vi "tcplink-client -- test.vi"() -> ()   [LabVIEW 2020]
uses:
  publisher action.ctl
  sparkle.ctl
panel:
  in  "millisecond multiple":u32=100
  in  "Stop":bool
  out "Gamma":dbl
  out "frequency":dbl
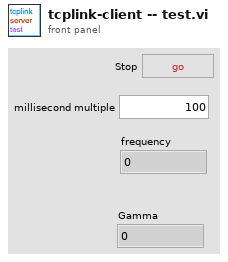
[diagram p1: front panel]
types:
  T1 = typedef "publisher action.ctl" = enum16{"set", "get", "init", "check"}
  T2 = typedef "sparkle.ctl" = cluster{"units":string, "data":dbl}
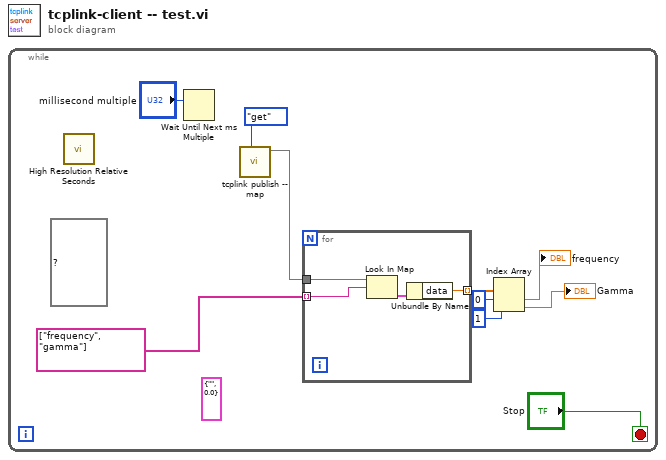
[diagram p0: block diagram]
diagram:
  n1 = while {
    stop <- "Stop" stop-if-true
    (unwired) T2 {"units"="", "data"=0.0} ("sparkle")
    (unwired) map{string, T2} {} ("sparkle map IN")
    n2 = call <vilib>:"High Resolution Relative Seconds.vi"() -> ()  [unwired: 1 out]
    n3 = Wait Until Next ms Multiple(millisecond multiple="millisecond multiple") -> ()  [unwired: 1 out]
    n4 = call "tcplink publish -- map.vi"("publisher action"=publisher_action."get") -> ("sparkle map OUT"=w6:map{string, T2})  [unwired: 10 in]
    n5 = for {
      tunnel: string[] ["frequency", "gamma"] ("string array IN") -> [w13] mode=indexing
      tunnel: w6 -> [w14]
      tunnel: [w11] -> w5 mode=indexing
      n6 = Look In Map(map=w14, key=w13) -> (value=w12:T2)  [unwired: 1 in, 1 out]
      n7 = Unbundle By Name(w12) -> ("data"=w11:dbl)
    }
    n8 = Index Array(array=w5, index #1=0 ("index"), index #2=1 ("index")) -> (element #1=→"frequency":dbl, element #2=→"Gamma":dbl)
  }
